vi "Destroy User Event - EHL Stop.vi"(8 "error in":errorcluster, 11 "User Event":refnum<user-event>) -> (0 "error out":errorcluster)   [LabVIEW 2016, in "User Event - EHL Stop.lvlib"]
doc: "Destroys the user event"
uses:
  User Event - EHL Stop.lvlib
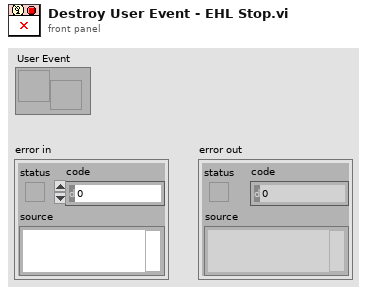
[diagram p1: front panel]
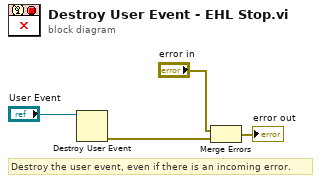
[diagram p0: block diagram]
diagram:
  # "Destroy the user event, even if there is an incoming error."
  n1 = Destroy User Event(user event="User Event") -> (error out=w3:errorcluster)  [unwired: 1 in]
  n2 = Merge Errors("error in", w3) -> (→"error out":errorcluster)
